vi "Calc Texel Colour.vi"(9 "Texture":T1, 10 "Texel Start":T3, 11 "Texel Delta Per Pixel in":T3) -> (2 "Texel Delta Per Pixel out":T3, 3 "Colour":u32)   [LabVIEW 2020, in "Raster (FPGA).lvlib"]
uses:
  Raster (FPGA).lvlib
  Rectangle Dimensions.ctl
  Texture.ctl
  Point 2D (SGL).ctl
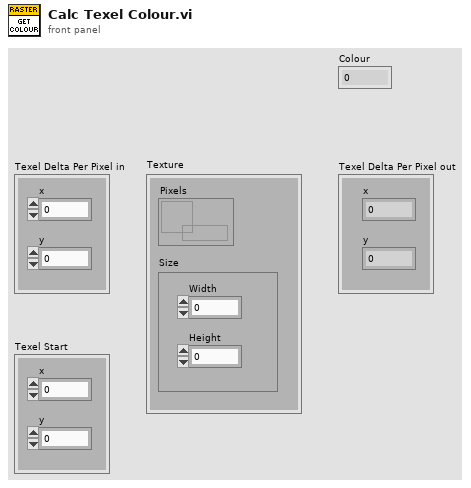
[diagram p1: front panel]
types:
  T1 = typedef "Raster (FPGA).lvlib/Texture.ctl" = cluster{"Pixels":refnum<data-value>, "Size":T2}
  T2 = typedef "Raster (FPGA).lvlib/Rectangle Dimensions.ctl" = cluster{"Width":u32, "Height":u32}
  T3 = typedef "Raster (FPGA).lvlib/Point 2D (SGL).ctl" = cluster{"x":sgl, "y":sgl}
  T4 = typedef "Raster (FPGA).lvlib/Point 2D (I32).ctl" = cluster{"x":i32, "y":i32}
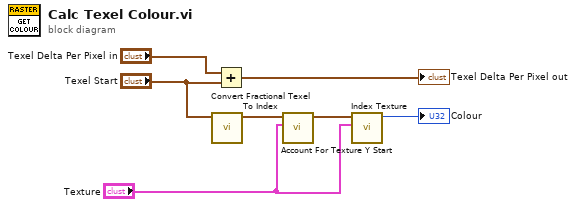
[diagram p0: block diagram]
diagram:
  n1 = call "Convert Fractional Texel To Index.vi"("Texel Start"="Texel Start") -> ("Texel As Pixel"=w7:T4)  [unwired: 10 in]
  n2 = Add(x="Texel Delta Per Pixel in", y="Texel Start") -> (x+y=→"Texel Delta Per Pixel out":T3)
  n3 = call "Account For Texture Y Start.vi"("Texture"="Texture", "Point"=w7) -> ("Point In Texture"=w5:T4)  [unwired: 9 in]
  n4 = call "Index Texture.vi"("Texture"="Texture", "Point In Texture"=w5) -> ("Colour"=→"Colour":u32)  [unwired: 9 in]
